vi "34401 - Find Range.vi"(0 "address":string, 5 "Number to Range (0.00)":ext format="%.10f", 9 "Numeric Data (Empty)":string, 11 "error in (no error)":errorcluster) -> (4 "dup address":string, 6 "Range Found":bool, 8 "Ranged Number":dbl format="%.7f", 10 "Index":dbl format="%.2f", 15 "error out":errorcluster)   [LabVIEW 2014]
doc: "Takes a given value and determines if the value belongs to a specified array of discrete numbers."
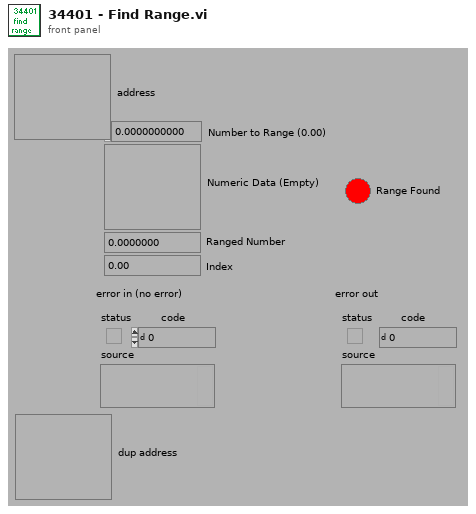
[diagram p1: front panel]
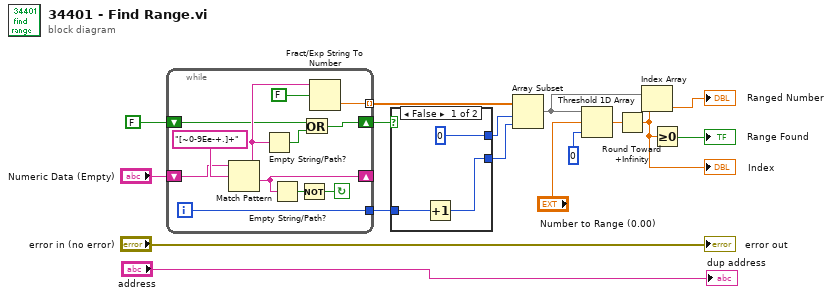
[diagram p0: block diagram]
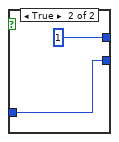
[diagram p2: hidden frame]
diagram:
  n1 = while {
    tunnel: [w23] -> w12 mode=indexing
    tunnel: [w21] -> w7
    shift-left: "Numeric Data (Empty)" -> [w27]
    shift-right: [w24] -> _
    shift-left: FALSE -> [w18]
    shift-right: [w19] -> w6
    i -> [w21]
    stop <- w25 continue-if-true
    n2 = Match Pattern(string=w27, regular expression="[~0-9Ee-+.]+") -> (before substring=w22:string, after substring=w24:string)  [unwired: 1 in, 2 out]
    n3 = Empty String/Path?(string/path=w22) -> (empty?=w20:bool)
    n4 = Empty String/Path?(string/path=w24) -> (empty?=w26:bool)
    n5 = Not(x=w26) -> (.not. x?=w25:bool)
    n6 = Or(x=w18, y=w20) -> (x .or. y?=w19:bool)
    n7 = Fract/Exp String To Number(use system decimal point (T)=FALSE, string=w22) -> (number=w23:dbl)  [unwired: 2 in, 1 out]
  }
  n8 = case shown="False" w6 {
    tunnel: [w29 w32] -> w8
    tunnel: [0 1] -> w9
    tunnel: w7 -> [w30 w32]
    frame False {
      n9 = Increment(x=w30) -> (x+1=w29:i32)
    }
    frame True {
    }
  }
  n10 = Array Subset(array=w12, index=w9, length=w8) -> (w11:dbl[])
  n11 = Threshold 1D Array(1:0, 2:"Number to Range (0.00)", 3:w11) -> (0:w5:dbl)
  n12 = Round Toward +Infinity(x=w5) -> (ceil(x): smallest int >= x=w4:dbl)
  "Index" <- w4
  n13 = Index Array(array=w11, index=w4) -> (element=→"Ranged Number":dbl)
  n14 = Greater Or Equal To 0?(x=w4) -> (x >= 0?=→"Range Found":bool)
  "error out" <- "error in (no error)"
  "dup address" <- "address"
